vi "After TS Config Tasks.vi"(8 "error in":errorcluster, 11 "DeepU Test Stand in":refnum<class "DeepU Test Stand.lvclass">) -> (0 "error out":errorcluster, 3 "DeepU Test Stand out":refnum<class "DeepU Test Stand.lvclass">)   [LabVIEW 2019, in "Test Stands.lvlib" / "DeepU Test Stand.lvclass"]
uses:
  DeepU Test Stand.lvclass
  Generic Test Stand/TS Panel Method.ctl
  Generic Test Stand/Generic Test Stand.lvclass
  Results/DeepU Results/DeepU Results.lvclass
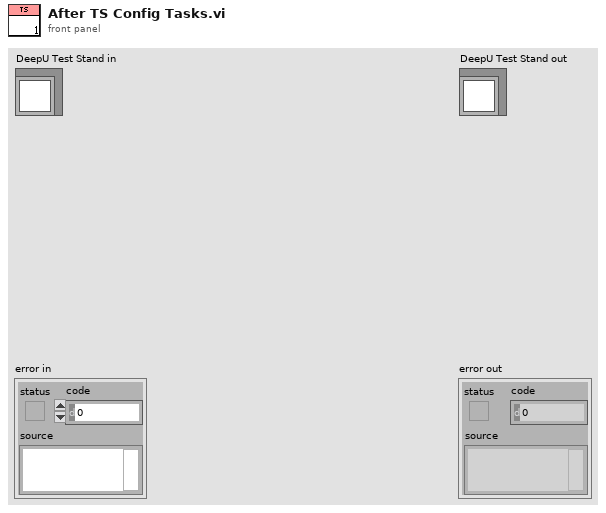
[diagram p1: front panel]
types:
  T1 = typedef "Generic Test Stand.lvclass/TS Panel Method.ctl" = enum16{"Send to Panel", "Receive from Panel", "Update Panel View"}
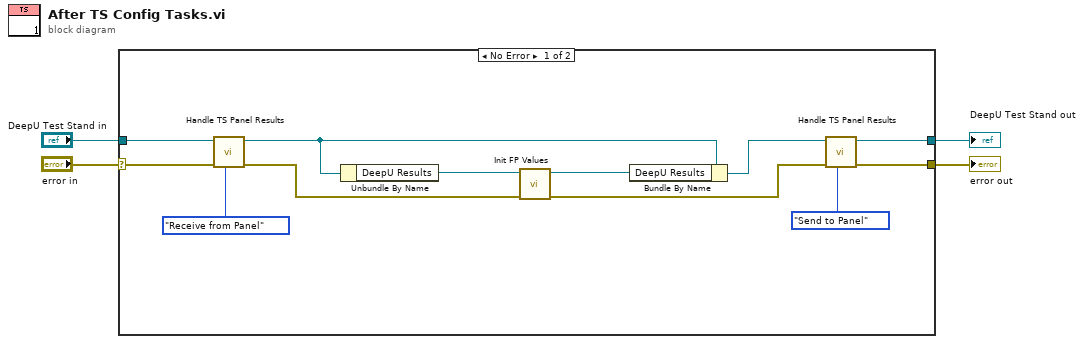
[diagram p0: block diagram]
diagram:
  n1 = case shown="No Error" "error in" {
    selector: "error in" -> [w8 w18]
    tunnel: [w5 w18] -> w4
    tunnel: [w15 w17] -> w3
    tunnel: "DeepU Test Stand in" -> [w16 w17]
    frame No Error {
      n2 = call-dynamic "Handle TS Panel Results.vi"("Method"=TS_Panel_Method."Receive from Panel", "error in"=w8, "DeepU Test Stand in"=w16) -> ("error out"=w7:errorcluster, "DeepU Test Stand out"=w12:refnum<class "DeepU Test Stand.lvclass">)  [unwired: 7 in]
      n3 = Unbundle By Name(w12) -> ("DeepU Results"=w11:refnum<class "DeepU Results.lvclass">)
      n4 = call "Init FP Values.vi"("error in (no error)"=w7, "DeepU Results in"=w11) -> ("error out"=w6:errorcluster, "DeepU Results out"=w9:refnum<class "DeepU Results.lvclass">)  [unwired: 8 in]
      n5 = Bundle By Name(cluster=w12, "DeepU Results"=w9) -> (w10:refnum<class "DeepU Test Stand.lvclass">)
      n6 = call-dynamic "Handle TS Panel Results.vi"("Method"=TS_Panel_Method."Send to Panel", "error in"=w6, "DeepU Test Stand in"=w10) -> ("error out"=w5:errorcluster, "DeepU Test Stand out"=w15:refnum<class "DeepU Test Stand.lvclass">)  [unwired: 7 in]
    }
    frame Error {
    }
  }
  "error out" <- w4
  "DeepU Test Stand out" <- w3
